vi "Get Sensor Mode.vi"(8 "error in (no error)":errorcluster, 11 "FW102C in":i32) -> (0 "error out":errorcluster, 2 "Sensor Mode":T1(ring), 3 "FW102C out":i32)   [LabVIEW 2015, in "Thorlabs_FW102C.lvlib"]
uses:
  Thorlabs_FW102C.lvlib
  <instrlib>/Thorlabs_FW102C/Library/FilterWheel102_win64.dll
  Library/FilterWheel102_win32.dll
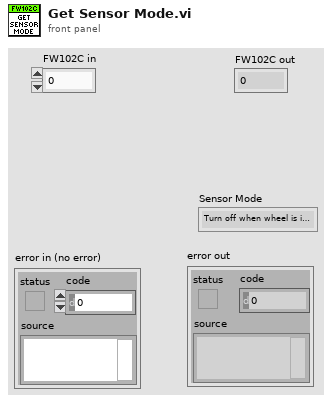
[diagram p1: front panel]
types:
  T1 = enum16{"Turn off when wheel is idle to eliminate stray light", "Remain active"}
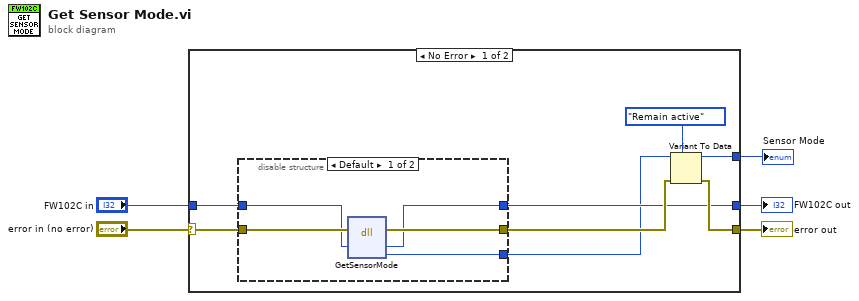
[diagram p0: block diagram]
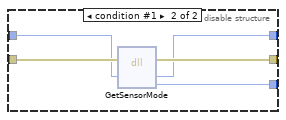
[diagram p2: hidden frame]
diagram:
  n1 = case shown="No Error" "error in (no error)" {
    selector: "error in (no error)" -> [w10 w24]
    tunnel: [w12 w24] -> w5
    tunnel: "FW102C in" -> [w8 w25]
    tunnel: [w7 w25] -> w2
    tunnel: [w13 _] -> w1
    frame No Error {
      n2 = disable-structure shown="Default" {
        disable-tunnel: w10 -> [w18 w23]
        disable-tunnel: [w17 w22] -> w9
        disable-tunnel: w8 -> [w16 w21]
        disable-tunnel: [w15 w20] -> w7
        disable-tunnel: [w14 w19] -> w6
        frame condition #0 (active) {
          n3 = dll-call lib="C:/Users/bspok/Desktop/AppNotes_FW102C_v400/AppNotes_FW102C/LabVIEW/Thorlabs_FW102C/Library/FilterWheel102_win32.dll" fn="GetSensorMode"(error in=w18, "hdl"=w16) -> (error out=w17:errorcluster, "hdl"=w15:i32, "sensor mode"=w14:i32)  [unwired: 4 in, 1 out]
        }
        frame condition #1 {
          n4 = dll-call lib="D:/Program Files/National Instruments/LabVIEW 2011/instr.lib/Thorlabs_FW102C/Library/FilterWheel102_win64.dll" fn="GetSensorMode"(error in=w23, "hdl"=w21) -> (error out=w22:errorcluster, "hdl"=w20:i32, "sensor mode"=w19:i32)  [unwired: 4 in, 1 out]
        }
      }
      n5 = Variant To Data(error in=w9, type=T1."Remain active" ("Sensor Mode"), Variant=w6) -> (data=w13:T1, error out=w12:errorcluster)
    }
    frame Error {
    }
  }
  "error out" <- w5
  "FW102C out" <- w2
  "Sensor Mode" <- w1
